vi "testRotUk.vi"(8 "error in (no error)":errorcluster) -> (0 "error out":errorcluster)   [LabVIEW 2016]
doc: "Test the rotation of uk."
uses:
  ZTAAC/ZTAAC.lvclass
  CamRot/CamRot.lvclass
  MatOper/getSubArray1D.vi
  <vilib>/addons/_JKI Toolkits/Caraya/classes/Test/Test.lvclass
  <vilib>/addons/_JKI Toolkits/Caraya/classes/Assert/Assert.lvclass
  MatOper/MatOper.lvclass
panel:
  in  "CamRot.lvclass":refnum<class "CamRot.lvclass">
  in  "ZTAAC.lvclass":refnum<class "ZTAAC.lvclass">
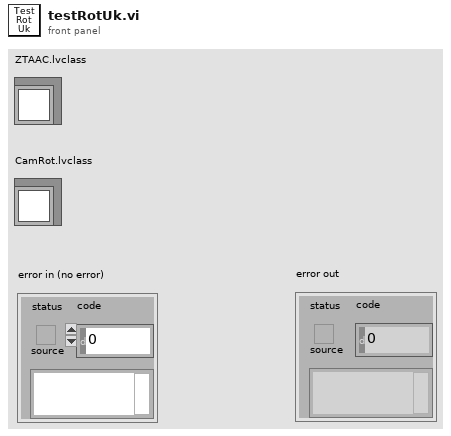
[diagram p1: front panel]
types:
  T1 = cluster{"M2 Hexapod":bool[], "Cam Hexapod ":bool[], "M1M3 Bending Mode":bool[], "M2 Bending Mode":bool[]}
  T2 = typedef "OfcFunc.lvlib/InstName.ctl" = enum16{"lsst", "comcam"}
  T3 = cluster{"Config Dir":path, "Inst Name":T2, "OptStateEsti Config File Name":string, "Mapping File Name":string, "Wavelength Table":string, "Intrinc Zk File Name":string, "y2 Corection File Name":string, "Index DOF File Name":string, "OptCtrl Config File Name":string, "State 0 File Name":string, "Weighting File Name":string, "PSSN Alpha File Name":string, "Authority Files":cluster{"Rigid Body Stroke File":string, "M1M3 Subsystem":cluster{"Mirror":string, "Actuatro Force File":string}, "M2 Subsystem":cluster{"Mirror":string, "Actuatro Force File":string}, "Num of Bending Mode":i32}, "Sensor Id to Name File Name":string, "Truncation Threshold":dbl, "Default Gain":dbl, "FWHM Threshold (arcsec)":dbl}
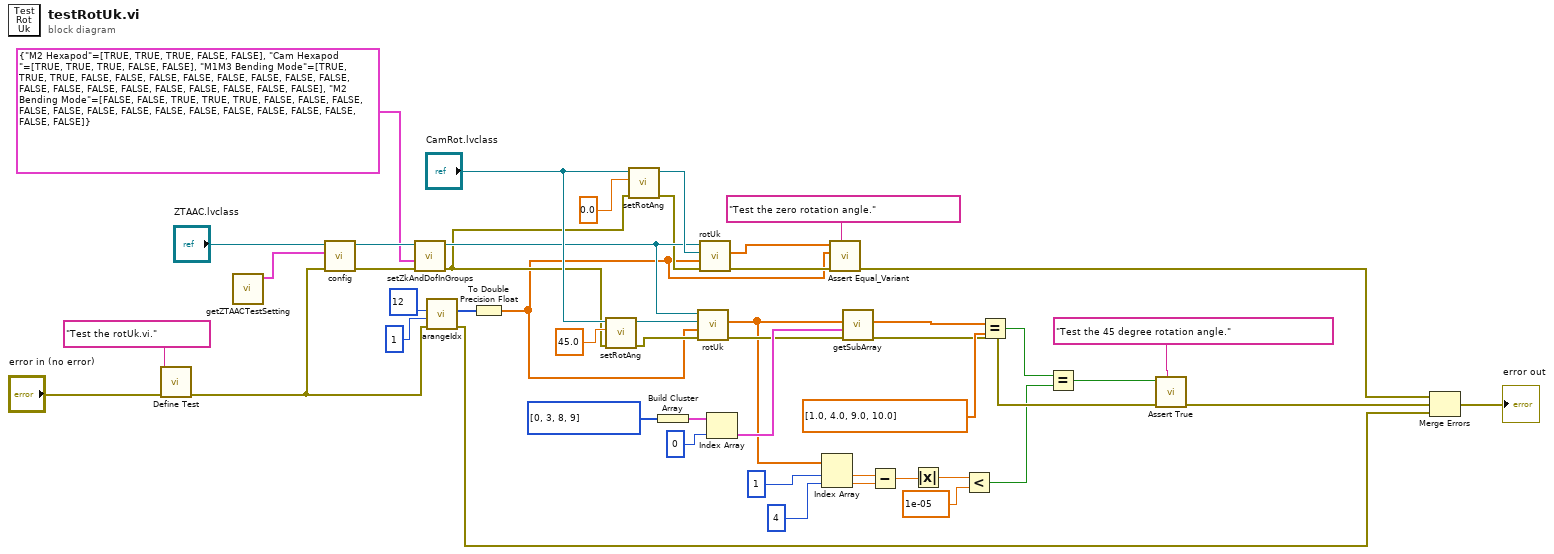
[diagram p0: block diagram]
diagram:
  n1 = call <vilib>:"Define Test.vi"("error in (no error)"="error in (no error)", "Label (VI Title)"="Test the rotUk.vi.") -> ("error out"=w3:errorcluster)  [unwired: 9 in]
  n2 = call "getZTAACTestSetting.vi"() -> ("Test Setting"=w1:T3)  [unwired: 11 in]
  n3 = call "config.vi"("error in (no error)"=w3, "ZTAAC Configuration"=w1, "ZTAAC in"="ZTAAC.lvclass") -> ("error out"=w34:errorcluster, "ZTAAC out"=w47:refnum<class "ZTAAC.lvclass">)  [unwired: 7 in]
  n4 = call "setZkAndDofInGroups.vi"("error in (no error)"=w34, "DOF in Groups"=T1 {"M2 Hexapod"=[TRUE, TRUE, TRUE, FALSE, FALSE], "Cam Hexapod "=[TRUE, TRUE, TRUE, FALSE, FALSE], "M1M3 Bending Mode"=[TRUE, TRUE, TRUE, FALSE, FALSE, FALSE, FALSE, FALSE, FALSE, FALSE, FALSE, FALSE, FALSE, FALSE, FALSE, FALSE, FALSE, FALSE, FALSE, FALSE], "M2 Bending Mode"=[FALSE, FALSE, TRUE, TRUE, TRUE, FALSE, FALSE, FALSE, FALSE, FALSE, FALSE, FALSE, FALSE, FALSE, FALSE, FALSE, FALSE, FALSE, FALSE, FALSE]}, "ZTAAC in"=w47) -> ("error out"=w33:errorcluster, "ZTAAC out"=w37:refnum<class "ZTAAC.lvclass">)  [unwired: 7 in]
  n5 = call "arangeIdx.vi"("error in (no error)"=w3, "Offset"=1, "Number"=12) -> ("error out"=w2:errorcluster, "Idx Array"=w42:i32[])  [unwired: 6 in, 1 out]
  n6 = To Double Precision Float(number=w42) -> (double precision float=w28:dbl[])
  n7 = call "setRotAng.vi"("error in (no error)"=w33, "Rotation Angle in Deg"=45.0, "CamRot in"="CamRot.lvclass") -> ("error out"=w32:errorcluster, "CamRot out"=w38:refnum<class "CamRot.lvclass">)  [unwired: 7 in]
  n8 = call "setRotAng.vi"("error in (no error)"=w33, "Rotation Angle in Deg"=0.0, "CamRot in"="CamRot.lvclass") -> ("error out"=w31:errorcluster, "CamRot out"=w44:refnum<class "CamRot.lvclass">)  [unwired: 7 in]
  n9 = Build Cluster Array(i32[] [0, 3, 8, 9]) -> (w26:cluster{i32[]}[])
  n10 = call "rotUk.vi"("error in (no error)"=w32, "uk Array"=w28, "CamRot in"=w38, "ZTAAC in"=w37) -> ("error out"=w22:errorcluster, "Rotated uk Array"=w15:dbl[])  [unwired: 5 in, 1 out]
  n11 = call "rotUk.vi"("error in (no error)"=w31, "uk Array"=w28, "CamRot in"=w44, "ZTAAC in"=w37) -> ("error out"=w30:errorcluster, "Rotated uk Array"=w29:dbl[])  [unwired: 5 in, 1 out]
  n12 = Index Array(array=w26, index=0) -> (element=w23:cluster{i32[]})
  n13 = Index Array(array=w15, index #1=1 ("index"), index #2=4 ("index")) -> (element #1=w9:dbl, element #2=w8:dbl)
  n14 = call <vilib>:"Assert Equal_Variant.vi"("Label"="Test the zero rotation angle.", "error in (no error)"=w30, "Y"=w28, "X"=w29) -> ("error out"=w17:errorcluster)  [unwired: 7 in]
  n15 = call-poly "getSubArray.vi"("error in (no error)"=w22, "Index Array Cluster"=w23, "1D Array"=w15) -> ("error out"=w10:errorcluster, "Sub-Array"=w21:dbl[])  [unwired: 6 in, 1 out]
  n16 = Subtract(x=w9, y=w8) -> (x-y=w7:dbl)
  n17 = Absolute Value(x=w7) -> (abs(x)=w6:dbl)
  n18 = Less?(x=w6, y=1e-05) -> (x < y?=w4:bool)
  n19 = Equal?(x=w21, y=dbl[] [1.0, 4.0, 9.0, 10.0]) -> (x = y?=w12:bool)
  n20 = Equal?(x=w12, y=w4) -> (x = y?=w11:bool)
  n21 = call <vilib>:"Assert True.vi"("Label"="Test the 45 degree rotation angle.", "error in (no error)"=w10, "True?"=w11) -> ("error out"=w16:errorcluster)  [unwired: 8 in]
  n22 = Merge Errors(w17, w16, w2) -> (→"error out":errorcluster)
